vi "Solve_residuals.vi"(7 "Alpha - Response Coefficients":cdb[][](array[numeric]), 8 "A-Base":cdb[][](array[numeric]), 9 "Alpha T'":cdb[][](array[numeric])) -> (0 "Epsilon":T1, 1 "Max Residual":dbl, 2 "W'":T1, 3 "|Epsilon/R||":T2, 4 "Sum of Squared Residuals":dbl, 5 "M":i32)   [LabVIEW 2010]
uses:
  <vilib>/Analysis/Matrix/Datatypes/RealMatrix.ctl
  <vilib>/Analysis/Matrix/Datatypes/ComplexMatrix.ctl
  <vilib>/Analysis/baseanly.llb/Complex A x B.vi
  <vilib>/Analysis/Matrix/Numeric/Multiply/Multiply - CM,C.vi
  <vilib>/Analysis/baseanly.llb/Complex Inverse Matrix.vi
  <vilib>/Analysis/Matrix/Numeric/Add/Add - CM,CM.vi
  <vilib>/Analysis/Matrix/Numeric/Conversions/Matrix To Array - CM.vi
  <vilib>/Analysis/Matrix/Numeric/Complex/Complex To Polar - CM.vi
  <vilib>/Analysis/NI_AALBase.lvlib
  <vilib>/Analysis/Matrix/NI_Matrix.lvlib
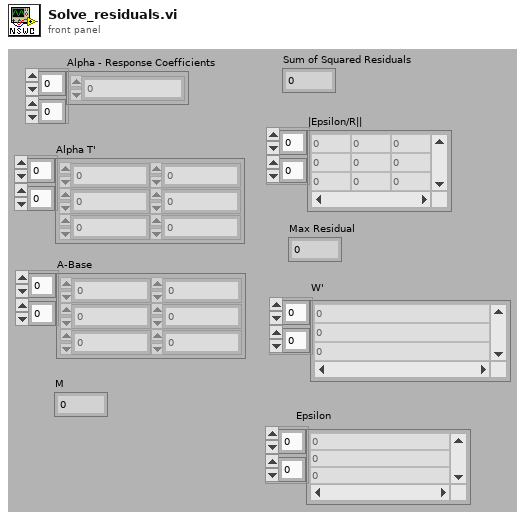
[diagram p1: front panel]
types:
  T1 = typedef "NI_Matrix.lvlib/ComplexMatrix.ctl" = cdb[][]
  T2 = typedef "NI_Matrix.lvlib/RealMatrix.ctl" = dbl[][]
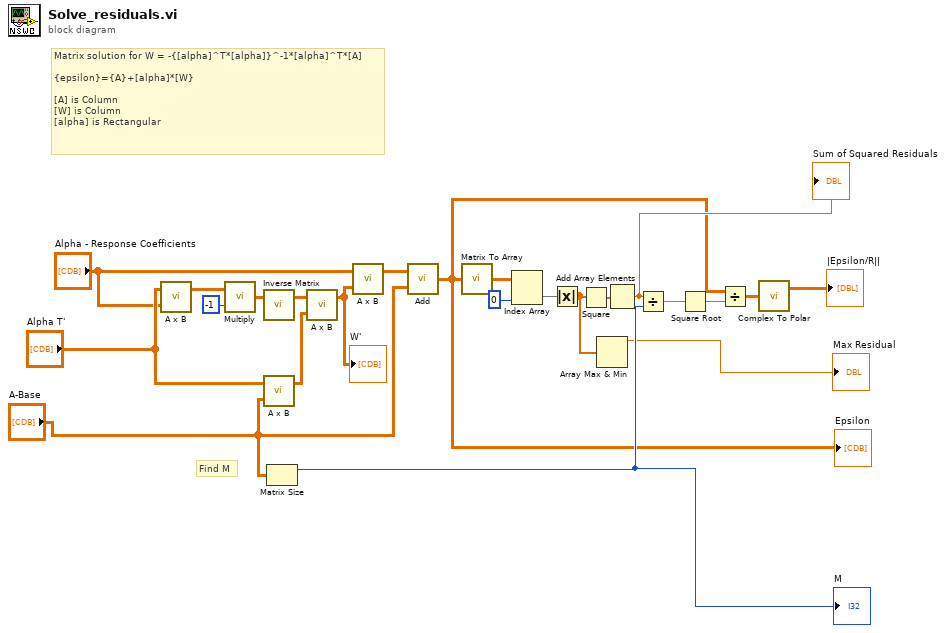
[diagram p0: block diagram]
diagram:
  # "Find M"
  # "Matrix solution for W = -{[alpha]^T*[alpha]}^-1*[alpha]^T*[A]\n\n{epsilon}={A}+[alpha]*[W}\n\n[A] is Column\n[W] is Column\n[alpha] is Rectangular"
  n1 = call-poly <vilib>:"A x B.vi"("B"="Alpha - Response Coefficients", "A"="Alpha T'") -> ("A x B"=w19:T1)  [unwired: 1 out]
  n2 = call-poly <vilib>:"Multiply.vi"("Complex Scalar c"=-1, "Complex Matrix A"=w19) -> ("A * c"=w20:T1)
  n3 = call-poly <vilib>:"Inverse Matrix.vi"("Input Matrix"=w20) -> ("Inverse Matrix"=w21:T1)  [unwired: 1 in, 1 out]
  n4 = call-poly <vilib>:"A x B.vi"("B"="A-Base", "A"="Alpha T'") -> ("A x B"=w17:T1)  [unwired: 1 out]
  n5 = Matrix Size(0:"A-Base") -> (1:w8:i32)  [unwired: 1 out]
  "M" <- w8
  n6 = call-poly <vilib>:"A x B.vi"("B"=w17, "A"=w21) -> ("A x B"=w23:T1)  [unwired: 1 out]
  "W'" <- w23
  n7 = call-poly <vilib>:"A x B.vi"("B"=w23, "A"="Alpha - Response Coefficients") -> ("A x B"=w16:T1)  [unwired: 1 out]
  n8 = call-poly <vilib>:"Add.vi"("Complex Matrix B"="A-Base", "Complex Matrix A"=w16) -> ("A + B"=w3:T1)
  "Epsilon" <- w3
  n9 = call-poly <vilib>:"Matrix To Array.vi"("Complex Matrix"=w3) -> ("Complex 2D Array"=w15:cdb[][])
  n10 = Index Array(array=w15, index (col)=0 ("disabled index (col)")) -> (element=w4:cdb[])  [unwired: 1 in]
  n11 = Absolute Value(x=w4) -> (abs(x)=w2:dbl[])
  n12 = Square(x=w2) -> (x^2=w13:dbl[])
  n13 = Array Max & Min(array=w2) -> (max value=→"Max Residual":dbl)  [unwired: 3 out]
  n14 = Add Array Elements(numeric array=w13) -> (sum=w12:dbl)
  "Sum of Squared Residuals" <- w12
  n15 = Divide(x=w12, y=w8) -> (x/y=w11:dbl)
  n16 = Square Root(x=w11) -> (sqrt(x)=w10:dbl)
  n17 = Divide(x=w3, y=w10) -> (x/y=w7:T1)
  n18 = call-poly <vilib>:"Complex To Polar.vi"("Complex Matrix r*e^iQ"=w7) -> ("Modulus r"=→"|Epsilon/R||":T2)  [unwired: 1 out]
